vi "main.vi"() -> ()   [LabVIEW 2015]
uses:
  global.vi
panel:
  in  "Aircraft 1 crashed? 2":bool
  in  "Aircraft 1 crashed?":bool
  in  "Center on Aircraft":enum32{"OFF", "Aircraft 1", "Aircraft 2"}(radio)
  in  "Zoom to Fit":bool
  out "URL":string
  in  "Aircraft 2":bool=TRUE
  in  "Aircraft 1":bool=TRUE
  in  "stop":bool
  in  "WebBrowser":refnum<k7>(container)
  # "Show:"
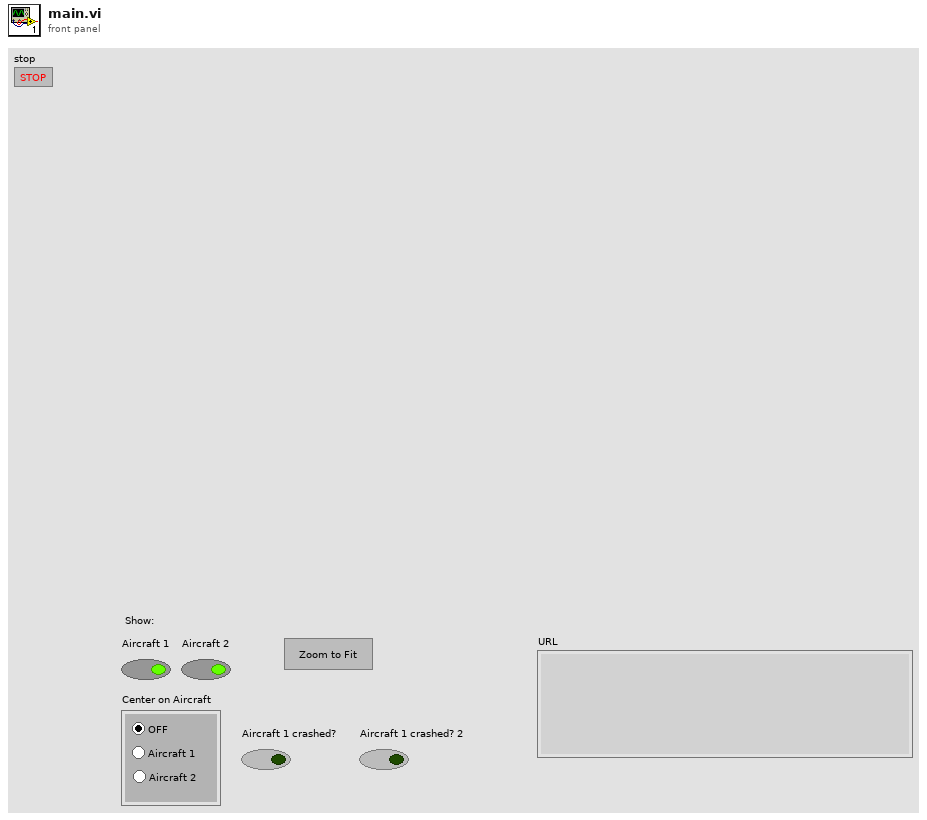
[diagram p1: front panel]
types:
  T1 = cluster{"Airspeed":dbl, "Altitude":dbl, "Vertical Speed":dbl, "Pitch":dbl, "Roll":dbl, "Heading":dbl, "Turn Indicator":dbl, "Latitude":dbl, "Longitude":dbl, "pilot g":dbl, "view number":i16, "fov":dbl, "view heading":dbl, "view pitch":dbl, "game width":i16, "game height":i16}
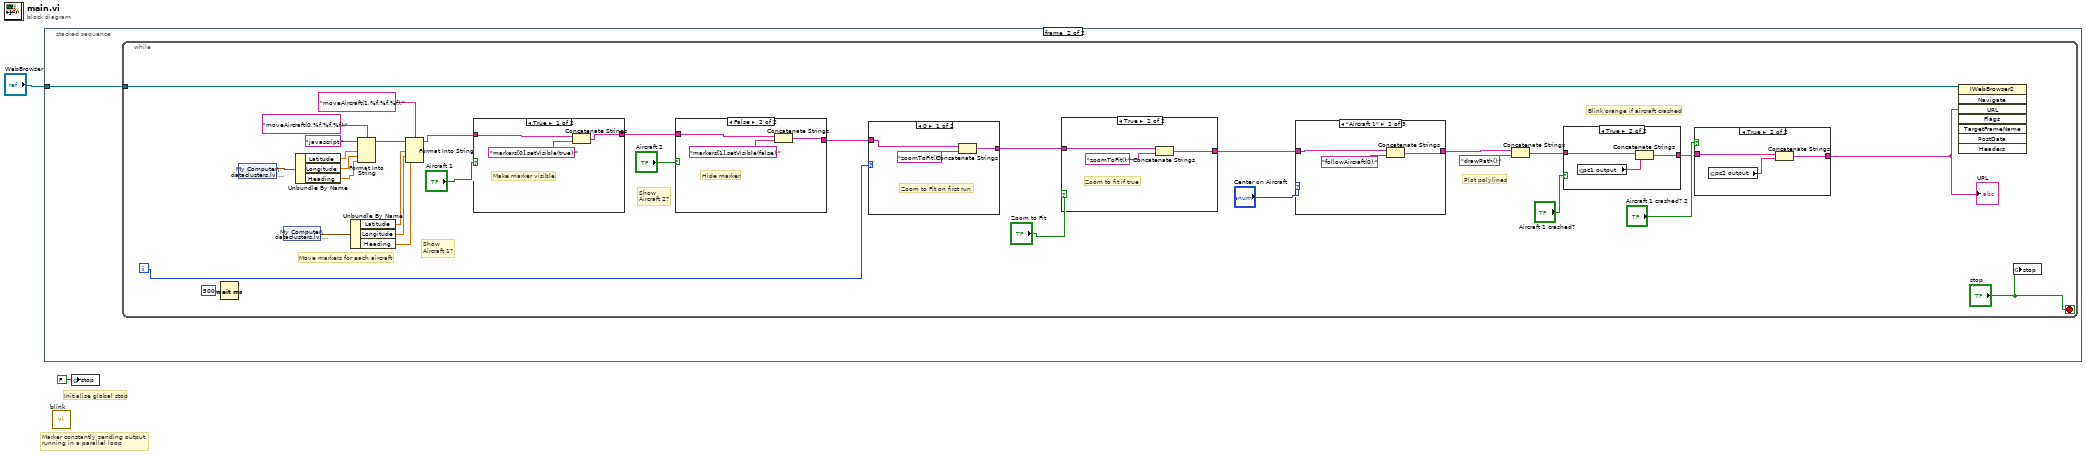
[diagram p0: block diagram]
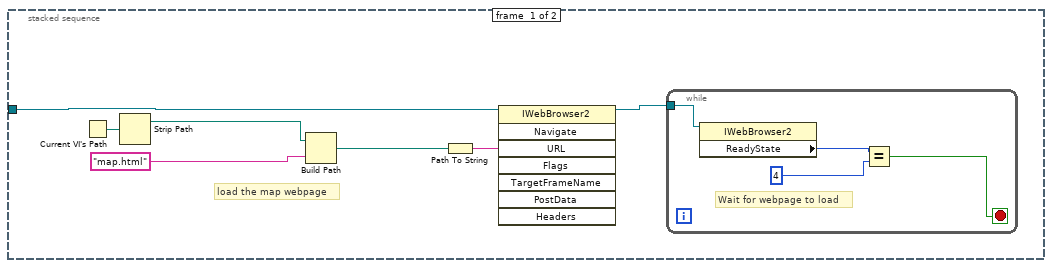
[diagram p2: hidden frame]
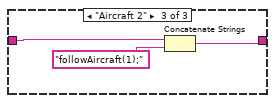
[diagram p6: hidden frame]
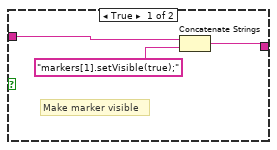
[diagram p9: hidden frame]
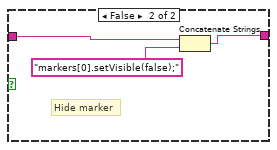
[diagram p10: hidden frame]
diagram:
  # "Initialise global stop"
  # "Marker constantly sending output,\nrunning in a parallel loop"
  n1 = stacked-sequence {
    tunnel: "WebBrowser" -> [w4 w14]
    frame #0 {
      # "load the map webpage"
      n2 = Current VI's Path() -> (path=w9:path)
      n3 = Strip Path(path=w9) -> (stripped path=w8:path)  [unwired: 1 out]
      n4 = Build Path(base path=w8, name or relative path="map.html") -> (appended path=w6:path)
      n5 = Path To String(path=w6) -> (string=w5:string)
      n6 = invoke class="IWebBrowser2" method="Navigate"(reference=w4, "URL"=w5) -> (reference out=w3:refnum<k7>)  [unwired: 6 in, 7 out]
      n7 = while {
        tunnel: w3 -> [w13]
        stop <- w10 stop-if-true
        # "Wait for webpage to load"
        n8 = property class="IWebBrowser2"(reference=w13) -> ("ReadyState"=w12:i32)  [unwired: 1 in, 2 out]
        n9 = Equal?(x=w12, y=4) -> (x = y?=w10:bool)
      }
    }
    frame #1 {
      n10 = while {
        tunnel: w14 -> [w45]
        i -> [w21]
        stop <- "stop" stop-if-true
        # "Blink orange if aircraft crashed"
        # "Plot polylines"
        # "Show\nAircraft 1?"
        # "Show\nAircraft 2?"
        # "Move markers for each aircraft"
        n11 = Wait (ms)(milliseconds to wait=u32 500) -> ()  [unwired: 1 out]
        n12 = shared-variable "My Computer\\dataclusters.lvlib\\pc1"() -> (w43:T1)  [unwired: 1 in, 1 out]
        n13 = shared-variable "My Computer\\dataclusters.lvlib\\pc2"() -> (w41:T1)  [unwired: 1 in, 1 out]
        n14 = Unbundle By Name(w43) -> ("Latitude"=w42:dbl, "Longitude"=w40:dbl, "Heading"=w22:dbl)
        n15 = Unbundle By Name(w41) -> ("Latitude"=w38:dbl, "Longitude"=w37:dbl, "Heading"=w23:dbl)
        n16 = Format Into String(format string="moveAircraft(0,%f,%f,%f);", initial string="javascript:", w42, w40, w22) -> (resulting string=w39:string)  [unwired: 1 in, 1 out]
        n17 = Format Into String(format string="moveAircraft(1,%f,%f,%f);", initial string=w39, w38, w37, w23) -> (resulting string=w34:string)  [unwired: 1 in, 1 out]
        n18 = case shown="True" "Aircraft 1" {
          tunnel: w34 -> [w78 w81]
          tunnel: [w76 w79] -> w32
          frame True {
            # "Make marker visible"
            n19 = Concatenate Strings(w78, "markers[0].setVisible(true);" ("string")) -> (w76:string)
          }
          frame False {
            # "Hide marker"
            n20 = Concatenate Strings(w81, "markers[0].setVisible(false);" ("string")) -> (w79:string)
          }
        }
        n21 = case shown="False" "Aircraft 2" {
          tunnel: w32 -> [w72 w75]
          tunnel: [w70 w73] -> w30
          frame True {
            # "Make marker visible"
            n22 = Concatenate Strings(w72, "markers[1].setVisible(true);" ("string")) -> (w70:string)
          }
          frame False {
            # "Hide marker"
            n23 = Concatenate Strings(w75, "markers[1].setVisible(false);" ("string")) -> (w73:string)
          }
        }
        n24 = case shown="0" w21 {
          tunnel: w30 -> [w68 w69]
          tunnel: [w66 w69] -> w28
          frame 0 {
            # "Zoom to Fit on first run"
            n25 = Concatenate Strings(w68, "zoomToFit();" ("string")) -> (w66:string)
          }
          frame 1, Default {
            # "Otherwise, do nothing"
          }
        }
        n26 = case shown="True" "Zoom to Fit" {
          tunnel: w28 -> [w62 w64]
          tunnel: [w62 w63] -> w26
          frame False {
          }
          frame True {
            # "Zoom to fit if true"
            n27 = Concatenate Strings(w64, "zoomToFit();" ("string")) -> (w63:string)
          }
        }
        n28 = case shown="\"Aircraft 1\"" "Center on Aircraft" {
          tunnel: w26 -> [w55 w58 w61]
          tunnel: [w55 w56 w59] -> w25
          frame "OFF", Default {
          }
          frame "Aircraft 1" {
            n29 = Concatenate Strings(w58, "followAircraft(0);" ("string")) -> (w56:string)
          }
          frame "Aircraft 2" {
            n30 = Concatenate Strings(w61, "followAircraft(1);" ("string")) -> (w59:string)
          }
        }
        n31 = Concatenate Strings(w25, "drawPath();" ("string")) -> (w18:string)
        n32 = case shown="True" "Aircraft 1 crashed?" {
          tunnel: w18 -> [w51 w54]
          tunnel: [w51 w53] -> w16
          frame False {
          }
          frame True {
            n33 = global read "global.vi" "pc1 output"() -> (w52:string)
            n34 = Concatenate Strings(w54, w52) -> (w53:string)
          }
        }
        n35 = case shown="True" "Aircraft 1 crashed? 2" {
          tunnel: w16 -> [w47 w50]
          tunnel: [w47 w49] -> w15
          frame False {
          }
          frame True {
            n36 = global read "global.vi" "pc2 output"() -> (w48:string)
            n37 = Concatenate Strings(w50, w48) -> (w49:string)
          }
        }
        "URL" <- w15
        n38 = invoke class="IWebBrowser2" method="Navigate"(reference=w45, "URL"=w15) -> ()  [unwired: 6 in, 8 out]
        n39 = global write "global.vi" "stop"("stop") -> ()
      }
    }
  }
  n40 = call "blink.vi"() -> ()  [unwired: 5 in]
  n41 = global write "global.vi" "stop"(FALSE ("stop")) -> ()
